vi "TheSigTab.vi"() -> ()   [LabVIEW 2010]
uses:
  <vilib>/Addons/database/Connection.llb/Conn ObjectReference.ctl
  <vilib>/addons/database/NI_Database_API.lvlib
panel:
  in  "Tabs":T1(tab)=enum."Amp"
  in  "DateString":string caption="Формат Даты"
  in  "SigTypeList":string[][](table) caption="Типы выходных сигналов"
  in  "DevNo":u32 caption="Измеритель"
  in  "ObjList":string[][](table) caption="Список объектов и измерителей"
  in  "Connection":T2 caption="ODBC"
  in  "InterfaceInfo":T3
  out "DeviceReady":bool caption="Устройство готово"
  in  "BufRQCounter":i32 caption="Счётчик обращений"
  in  "Changed":bool caption="Настройки Изменены"
  out "data addr":u32 format="%x"
  out "sync addr":u32 format="%x"
  in  "BufSize":u32 caption="Размер буфера"
  in  "hIfc":u32 format="%x"
  in  "main_value":sgl[](array[numeric]) caption="Q(R50), мВ"
  in  "Q(R50)":sgl[](array[numeric]) caption="Q(R50), мВ"
  in  "QCalibr":i32=1000 caption="Тест. Заряд (пК)"
  in  "Mode":u16(ring)=1 caption="Умножение" items=["Единичное", "Диагональное", "Полное"]
  in  "MatrixCalibr":dbl[][](array[numeric])=[[1.0, 0.0, 0.0, 0.0], [0.0, 1.0, 0.0, 0.0], [0.0, 0.0, 1.0, 0.0], [0.0, 0.0, 0.0, 1.0]] caption="Коеффициенты градуировки ( пК / мВ )" format="%.3f"
  in  "SyncTag":i32=-1 caption="Привязка"
  in  "F0":dbl caption="Начальный сдвиг"
  in  "off_len":cluster{"offset":dbl, "length":dbl}[](array[cluster]) caption="Параметры окон"
  in  "Units":string[](array[string])=["%", "мВ", "Градусы", "атм"] caption="Ед.изм.(первый столбец)"
  in  "K":dbl[][](array[numeric]) caption="Коэффициенты усилителя" format="%.4f"
  in  "DAQParam":T4={"s_Type"=1, "FIFO"=2045, "IrqStep"=2045, "Pages"=401, "AutoInit"=1, "dRate"=1144.0, "dKadr"=0.0, "dScale"=0.0, "Rate"=0, "Kadr"=0, "Scale"=0, "FPDelay"=0, "SynchroType"=3, "SynchroSensitivity"=0, "SynchroMode"=0, "AdChannel"=1, "AdPorog"=0, "NCh"=5, "Chn"=[36, 32, 1, 2, 3, 0, 0, 0, 0, 0, 0, 0, 0, 0, 0, 0, 0, 0, 0, 0, 0, 0, 0, 0, 0, 0, 0, 0, 0, 0, 0, 0, 0, 0, 0, 0, 0, 0, 0, 0, 0, 0, 0, 0, 0, 0, 0, 0, 0, 0, 0, 0, 0, 0, 0, 0, 0, 0, 0, 0, 0, 0, 0, 0, 0, 0, 0, 0, 0, 0, 0, 0, 0, 0, 0, 0, 0, 0, 0, 0, 0, 0, 0, 0, 0, 0, 0, 0, 0, 0, 0, 0, 0, 0, 0, 0, 0, 0, 0, 0, 0, 0, 0, 0, 0, 0, 0, 0, 0, 0, 0, 0, 0, 0, 0, 0, 0, 0, 0, 0, 0, 0, 0, 0, 0, 0, 0, 0], "IrqEna"=1, "AdcEna"=1} caption="Настройки АЦП"
  in  "SigTable":T5(array[cluster]) caption="Таблица Входных Сигналов"
  in  "SigOut":string[][](table) caption="Сигналы этого измерителя"
  in  "Sig2Obj":string[](array[string]) caption="Объекты этого измерителя"
  in  "Imbalance":cdb[](array[numeric])=[0.0+0.0i, 0.0+0.0i, 0.0+0.0i, 0.0+0.0i, 0.0+0.0i] caption="Небаланс"
  in  "path":path=path "C:/Documents and Settings/Андрей/User/A_Stend/RW/tests/Ufft70.ini" caption="Файл конфигурации"
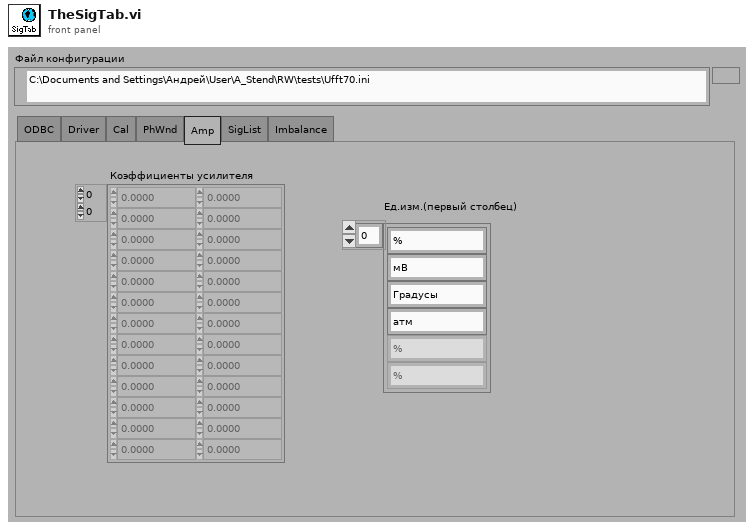
[diagram p1: front panel]
types:
  T1 = enum32{"ODBC", "Driver", "Cal", "PhWnd", "Amp", "SigList", "Imbalance"}
  T2 = typedef "NI_Database_API.lvlib/Conn ObjectReference.ctl" = refnum<k1>
  T3 = cluster{"DllVersion":u32, "InterfaceType":u32, "InterfaceInstance":u32, "ModuleHandle":u32, "ReadBuffersParsArray":cluster{"Buffer":i16[], "ReadOv":u32, "ReadEvent":u32}[], "WriteBuffersParsArray":cluster{"Buffer":i16[], "WriteOv":u32, "WriteEvent":u32}[]}
  T4 = cluster{"s_Type":u16, "FIFO":u16, "IrqStep":u16, "Pages":u16, "AutoInit":u16, "dRate":dbl, "dKadr":dbl, "dScale":dbl, "Rate":u16, "Kadr":u16, "Scale":u16, "FPDelay":u16, "SynchroType":u16, "SynchroSensitivity":u16, "SynchroMode":u16, "AdChannel":u16, "AdPorog":u16, "NCh":u16, "Chn":i32[], "IrqEna":u16, "AdcEna":u16}
  T5 = cluster{"Сигнал":string, "Тип":enum16{"Напряжение/Ток", "ЧР", "Температура", "Давление"}, "Object":string}[]
diagram:
